vi "N Channel 1 Sample - Auto Indexing.vi"() -> ()   [LabVIEW 2026, in "synnax_lib.lvlib"]
uses:
  lvproj/lvlib/synnax_lib.lvlib
  lvproj/lvlib/classes/Synnax Writer.lvclass
  lvproj/lvlib/classes/Client/Synnax Client.lvclass
  lvproj/lvlib/classes/Client/Private/synnax channel retrieve keys Array.vi
  lvproj/lvlib/classes/Writer/Private/synnax writer open Array.vi
  lvproj/lvlib/classes/Writer/Private/Writes/I32/Write NCh 1Samp (I32).vi
  lvproj/lvlib/typedefs/connection_config.ctl
panel:
  out "error out":errorcluster
  in  "Channels":string[](array[numeric])=["my_i32_ch1", "my_i32_ch2", "my_i32_ch3", "my_i32_ch4"]
  in  "Stop":bool
  in  "Connection Config":T1={"host"="localhost", "port"=9090, "username"="synnax", "password"="seldon"}
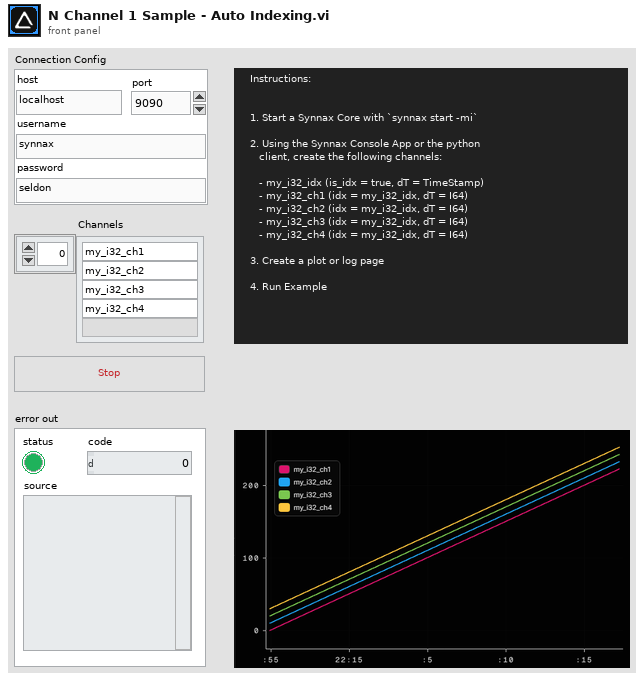
[diagram p1: front panel]
types:
  T1 = typedef "synnax_lib.lvlib/connection_config.ctl" = cluster{"host":string, "port":u16, "username":string, "password":string}
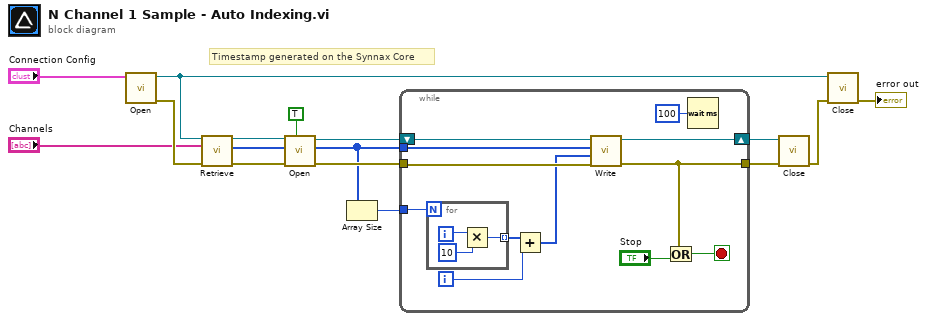
[diagram p0: block diagram]
diagram:
  # "Timestamp generated on the Synnax Core"
  n1 = call "Open.vi"("Connection Config"="Connection Config") -> ("error out"=w11:errorcluster, "Synnax Client out"=w13:refnum<class "Synnax Client.lvclass">)  [unwired: 9 in]
  n2 = call-poly "Retrieve.vi"("Synnax Client in"=w13, "channel names"="Channels", "error in"=w11) -> ("Synnax Client out"=w7:refnum<class "Synnax Client.lvclass">, "channel keys"=w6:u32[], "error out"=w15:errorcluster)  [unwired: 8 in, 2 out]
  n3 = call-poly "Open.vi"("auto_index (F)"=TRUE, "error in"=w15, "channels in"=w6, "Synnax Client in"=w7) -> ("error out"=w8:errorcluster, "channels out"=w4:u32[], "writer out"=w10:refnum<class "Synnax Writer.lvclass">)  [unwired: 5 in]
  n4 = Array Size(array=w4) -> (size(s)=w3:i32)
  n5 = while {
    shift-right: [w27] -> w9
    shift-left: w10 -> [w28]
    tunnel: w8 -> [w26]
    tunnel: [w17] -> w16
    tunnel: w4 -> [w22]
    tunnel: w3 -> [w21]
    i -> [w19]
    stop <- w18 stop-if-true
    n6 = for {
      N: w21 -> [_]
      tunnel: [w30] -> w24 mode=indexing
      i -> [w31]
      n7 = Multiply(x=w31, y=10) -> (x*y=w30:i32)
    }
    n8 = Add(x=w24, y=w19) -> (x+y=w20:i32[])
    n9 = call-poly "Write.vi"("error in"=w26, "data"=w20, "channels"=w22, "Writer"=w28) -> ("error out"=w17:errorcluster, "Writer Out"=w27:refnum<class "Synnax Writer.lvclass">)  [unwired: 6 in]
    n10 = Or(x=w17, y="Stop") -> (x .or. y?=w18:bool)
    n11 = Wait (ms)(milliseconds to wait=u32 100) -> ()  [unwired: 1 out]
  }
  n12 = call "Close.vi"("error in"=w16, "writer"=w9) -> ("error out"=w12:errorcluster)  [unwired: 9 in]
  n13 = call "Close.vi"("error in"=w12, "Synnax Client in"=w13) -> ("error out"=→"error out":errorcluster)  [unwired: 9 in]
